vi "configure.vi"(8 "error in (no error)":errorcluster, 9 "write enable":bool=TRUE, 11 "SMSD in":refnum<class "SMSD.lvclass">) -> (0 "error out":errorcluster, 3 "SMSD out":refnum<class "SMSD.lvclass">)   [LabVIEW 2021, in "SMSD.lvclass"]
uses:
  SMSD.lvclass
  D:/my_projects/projects/Algorithms/Labview/21/Modbus/MB_TCP2/MB_TCP.lvclass
  SMSD.lvclass/SMSD.ctl
  Ctl/ERROR_OR_COMMANT_Type.ctl
  MB_TCP.lvclass/MB_TCP.ctl
  NI_modbus_upd/TCP/TCP.lvclass/TCP.ctl
  SMSD_cmd_format.vi
  NI_modbus_upd/TCP/Protocol Read.vi
  NI_modbus_upd/TCP/Protocol Write.vi
  Data Access/Read TCP.vi
  SMSD_cmd_Data_format.vi
  SMSD_LAN_COMMAND.vi
  <vilib>/Utility/error.llb/Clear Errors.vi
  NI_modbus_upd/TCP/TCP.lvclass
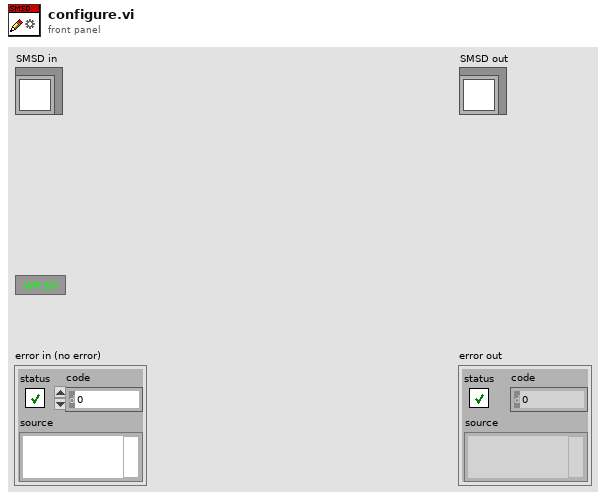
[diagram p1: front panel]
types:
  T1 = enum8{"CMD_PowerSTEP01_END", "CMD_PowerSTEP01_GET_SPEED", "CMD_PowerSTEP01_STATUS_IN_EVENT", "CMD_PowerSTEP01_SET_MODE", "CMD_PowerSTEP01_GET_MODE", "CMD_PowerSTEP01_SET_MIN_SPEED", "CMD_PowerSTEP01_SET_MAX_SPEED", "CMD_PowerSTEP01_SET_ACC", "CMD_PowerSTEP01_SET_DEC", "CMD_PowerSTEP01_SET_FS_SPEED", "CMD_PowerSTEP01_SET_MASK_EVENT", "CMD_PowerSTEP01_GET_ABS_POS", "CMD_PowerSTEP01_GET_EL_POS", "CMD_PowerSTEP01_GET_STATUS_AND_CLR", "CMD_PowerSTEP01_RUN_F", "CMD_PowerSTEP01_RUN_R", "CMD_PowerSTEP01_MOVE_F", "CMD_PowerSTEP01_MOVE_R", "CMD_PowerSTEP01_GO_TO_F", "CMD_PowerSTEP01_GO_TO_R", "CMD_PowerSTEP01_GO_UNTIL_F", "CMD_PowerSTEP01_GO_UNTIL_R", "CMD_PowerSTEP01_SCAN_ZERO_F", "CMD_PowerSTEP01_SCAN_ZERO_R", "CMD_PowerSTEP01_SCAN_LABEL_F", "CMD_PowerSTEP01_SCAN_LABEL_R", "CMD_PowerSTEP01_GO_ZERO", "CMD_PowerSTEP01_GO_LABEL", "CMD_PowerSTEP01_GO_TO", "CMD_PowerSTEP01_RESET_POS", "CMD_PowerSTEP01_RESET_POWERSTEP01", "CMD_PowerSTEP01_SOFT_STOP", "CMD_PowerSTEP01_HARD_STOP", "CMD_PowerSTEP01_SOFT_HI_Z", "CMD_PowerSTEP01_HARD_HI_Z", "CMD_PowerSTEP01_SET_WAIT", "CMD_PowerSTEP01_SET_RELE", "CMD_PowerSTEP01_CLR_RELE", "CMD_PowerSTEP01_GET_RELE", "CMD_PowerSTEP01_WAIT_IN0", "CMD_PowerSTEP01_WAIT_IN1", "CMD_PowerSTEP01_GOTO_PROGRAM", "CMD_PowerSTEP01_GOTO_PROGRAM_IF_IN0", "CMD_PowerSTEP01_GOTO_PROGRAM_IF_IN1", "CMD_PowerSTEP01_LOOP_PROGRAM", "CMD_PowerSTEP01_CALL_PROGRAM", "CMD_PowerSTEP01_RETURN_PROGRAM", "CMD_PowerSTEP01_START_PROGRAM_MEM0", "CMD_PowerSTEP01_START_PROGRAM_MEM1", "CMD_PowerSTEP01_START_PROGRAM_MEM2", "CMD_PowerSTEP01_START_PROGRAM_MEM3", "CMD_PowerSTEP01_STOP_PROGRAM_MEM", "CMD_PowerSTEP01_STEP_CLOCK", "CMD_PowerSTEP01_STOP_USB", "CMD_PowerSTEP01_GET_MIN_SPEED", "CMD_PowerSTEP01_GET_MAX_SPEED", "CMD_PowerSTEP01_GET_STACK", "CMD_PowerSTEP01_GOTO_PROGRAM_IF_ZERO", "CMD_PowerSTEP01_GOTO_PROGRAM_IF_IN_ZERO", "CMD_PowerSTEP01_WAIT_CONTINUE", "CMD_PowerSTEP01_SET_WAIT_2", "CMD_PowerSTEP01_SCAN_MARK2_F", "CMD_PowerSTEP01_SCAN_MARK2_R"}
  T2 = typedef "SMSD.lvclass/ERROR_OR_COMMANT_Type.ctl" = enum8{"OK", "OK_ACCESS", "ERROR_ACCESS", "ERROR_ACCESS_TIMEOUT", "ERROR_XOR", "ERROR_NO_COMMAND", "ERROR_LEN", "ERROR_RANGE", "ERROR_WRITE", "ERROR_READ", "ERROR_PROGRAMS", "ERROR_WRITE_SETUP", "NO_NEXT", "END_PROGRAMS", "COMMAND_GET_STATUS_IN_EVENT", "COMMAND_GET_MODE", "COMMAND_GET_ABS_POS", "COMMAND_GET_EL_POS", "COMMAND_GET_SPEED", "COMMAND_GET_MIN_SPEED", "COMMAND_GET_MAX_SPEED", "COMMAND_GET_STACK", "STATUS_RELE_SET", "STATUS_RELE_CLR"}
  T3 = cluster{"min_speed":u32, "max_speed":u32, "acc":u32, "dec":u32}
  T4 = typedef "SMSD.lvclass/MOTOR_PARAM.ctl" = cluster{"DRIVER_MODE":T5, "MOTOR_Type_42":T6, "MICROSTEPPING":T7, "WORK_CURRENT":T8, "STOP_CURRENT":T9}
  T5 = typedef "SMSD.lvclass/DRIVER_MODE.ctl" = enum16{"VOLTAGE", "CURRENT"}
  T6 = typedef "SMSD.lvclass/MOTOR_Type_42.ctl" = enum16{"Unknown", "FL42STH33-1334 1.8 deg", "FL42STH33-1334 0.9 deg", "FL42STH38-1206 0.9 deg", "FL42STH38-1684 1.8 deg", "FL42STH38-1684 0.9 deg", "FL42STH47-1206 1.8 deg", "FL42STH47-1684 1.8 deg", "FL42STH47-1684 0.9 deg", "FL42STH60-1206 1.8 deg", "FL42STH60-1206 0.9 deg", "FL57ST41-1564 1.8 deg", "FL57ST76-1006 1.8 deg", "FL57ST76-1506 1.8 deg", "FL57STH41-1006 1.8 deg", "FL57STH41-1006 0.9 deg", "FL57STH41-2804 1.8 deg", "FL57STH41-2804 0.9 deg", "FL57STH51-1006 1.8 deg", "FL57STH51-2804 1.8 deg", "FL57STH51-2804 0.9 deg", "FL57STH56-1006 1.8 deg", "FL57STH56-2006 1.8 deg", "FL57STH56-2804 1.8 deg", "FL57STH76-1006 1.8 deg", "FL57STH76-2804 1.8 deg", "FL57STH76-2804 0.9 deg", "FL60STH65-2008 1.8 deg parallel", "FL60STH65-2008 1.8 deg serial", "FL60STH86-2008 1.8 deg parallel", "FL60STH86-2008 1.8 deg serial", "FL86STH65-2808 1.8 deg parallel", "FL86STH65-2808 1.8 deg serial", "FL86STH80-4208 1.8 deg parallel", "FL86STH80-4208 1.8 deg serial", "FL86STH118-4208 1.8 deg parallel", "FL86STH118-4208 1.8 deg serial", "FL86STH156-4208 1.8 deg parallel", "FL86STH156-4208 1.8 deg serial", "ДШ3934-0,3А", "ДШ2851-0,7А", "ДШ4248-1,7A", "ДШ5776-3,0А", "ДШ57112-3,0А", "ДШ8665-3,0А", "ДШ8682-4,5А"}
  T7 = typedef "SMSD.lvclass/MICROSTEPPING.ctl" = enum16{"1", "1/2", "1/4", "1/8", "1/16", "1/32", "1/64", "1/128"}
  T8 = typedef "SMSD.lvclass/WORK_CURRENT.ctl" = enum16{"0.0A", "0.1A", "0.2A", "0.3A", "0.4A", "0.5A", "0.6A", "0.7A", "0.8A", "0.9A", "1.0A", "1.1A", "1.2A", "1.3A", "1.4A", "1.5A", "1.6A", "1.7A", "1.8A", "1.9A", "2.0A", "2.1A", "2.2A", "2.3A", "2.4A", "2.5A", "2.6A", "2.7A", "2.8A", "2.9A", "3.0A", "3.1A", "3.2A", "3.3A", "3.4A", "3.5A", "3.6A", "3.7A", "3.8A", "3.9A", "4.0A", "4.1A", "4.2A"}
  T9 = typedef "SMSD.lvclass/STOP_CURRENT.ctl" = enum16{"25%", "50%", "75%", "100%"}
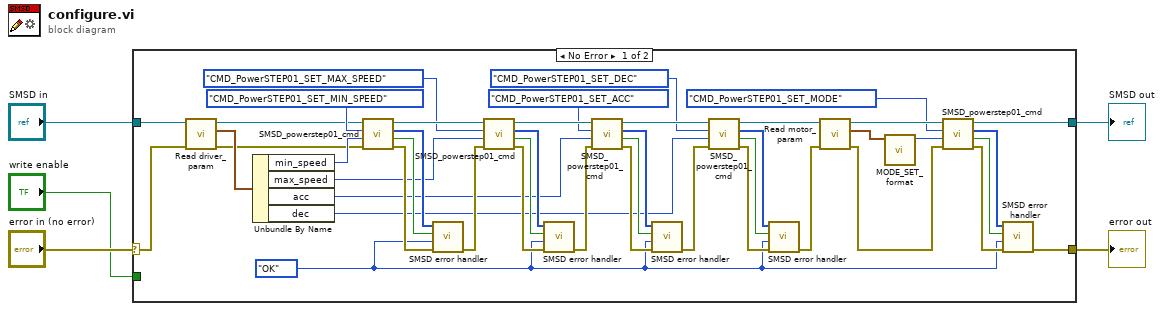
[diagram p0: block diagram]
diagram:
  n1 = case shown="No Error" "error in (no error)" {
    selector: "error in (no error)" -> [w6 w51]
    tunnel: [w12 w51] -> w3
    tunnel: [w10 w50] -> w4
    tunnel: "SMSD in" -> [w7 w50]
    tunnel: "write enable" -> [_ _]
    frame No Error {
      w11 = ERROR_OR_COMMANT_Type."OK" ("coerced x 2")
      n2 = call "Read driver_param.vi"("error in (no error)"=w6, "SMSD in"=w7) -> ("error out"=w45:errorcluster, "Driver_param"=w47:T3, "SMSD out"=w48:refnum<class "SMSD.lvclass">)  [unwired: 7 in]
      n3 = Unbundle By Name(w47) -> ("min_speed"=w46:u32, "max_speed"=w39:u32, "acc"=w29:u32, "dec"=w21:u32)
      n4 = call "SMSD_powerstep01_cmd.vi"("error in (no error)"=w45, "DATA (0)"=w46, "COMMAND (END)"=T1."CMD_PowerSTEP01_SET_MIN_SPEED", "SMSD in"=w48) -> ("error out"=w43:errorcluster, "timed out?"=w42:bool, "data"=w44:u8[], "SMSD out"=w41:refnum<class "SMSD.lvclass">)  [unwired: 4 in]
      n5 = call "SMSD error handler.vi"("error in (no error)"=w43, "correct answer (OK)"=w11, "timed out?"=w42, "data"=w44) -> ("error out"=w38:errorcluster)  [unwired: 7 in]
      n6 = call "SMSD_powerstep01_cmd.vi"("error in (no error)"=w38, "DATA (0)"=w39, "COMMAND (END)"=T1."CMD_PowerSTEP01_SET_MAX_SPEED", "SMSD in"=w41) -> ("error out"=w35:errorcluster, "timed out?"=w36:bool, "data"=w37:u8[], "SMSD out"=w30:refnum<class "SMSD.lvclass">)  [unwired: 4 in]
      n7 = call "SMSD error handler.vi"("error in (no error)"=w35, "correct answer (OK)"=w11, "timed out?"=w36, "data"=w37) -> ("error out"=w31:errorcluster)  [unwired: 7 in]
      n8 = call "SMSD_powerstep01_cmd.vi"("error in (no error)"=w31, "DATA (0)"=w29, "COMMAND (END)"=T1."CMD_PowerSTEP01_SET_ACC", "SMSD in"=w30) -> ("error out"=w34:errorcluster, "timed out?"=w33:bool, "data"=w32:u8[], "SMSD out"=w25:refnum<class "SMSD.lvclass">)  [unwired: 4 in]
      n9 = call "SMSD error handler.vi"("error in (no error)"=w34, "correct answer (OK)"=w11, "timed out?"=w33, "data"=w32) -> ("error out"=w24:errorcluster)  [unwired: 7 in]
      n10 = call "SMSD_powerstep01_cmd.vi"("error in (no error)"=w24, "DATA (0)"=w21, "COMMAND (END)"=T1."CMD_PowerSTEP01_SET_DEC", "SMSD in"=w25) -> ("error out"=w26:errorcluster, "timed out?"=w27:bool, "data"=w28:u8[], "SMSD out"=w20:refnum<class "SMSD.lvclass">)  [unwired: 4 in]
      n11 = call "SMSD error handler.vi"("error in (no error)"=w26, "correct answer (OK)"=w11, "timed out?"=w27, "data"=w28) -> ("error out"=w8:errorcluster)  [unwired: 7 in]
      n12 = call "Read motor_param.vi"("error in (no error)"=w8, "SMSD in"=w20) -> ("error out"=w9:errorcluster, "MOTOR_PARAM"=w19:T4, "SMSD out"=w15:refnum<class "SMSD.lvclass">)  [unwired: 7 in]
      n13 = call "MODE_SET_format.vi"("MOTOR_PARAM"=w19) -> ("Data"=w13:u32)  [unwired: 10 in]
      n14 = call "SMSD_powerstep01_cmd.vi"("error in (no error)"=w9, "DATA (0)"=w13, "COMMAND (END)"=T1."CMD_PowerSTEP01_SET_MODE", "SMSD in"=w15) -> ("error out"=w18:errorcluster, "timed out?"=w17:bool, "data"=w16:u8[], "SMSD out"=w10:refnum<class "SMSD.lvclass">)  [unwired: 4 in]
      n15 = call "SMSD error handler.vi"("error in (no error)"=w18, "correct answer (OK)"=w11, "timed out?"=w17, "data"=w16) -> ("error out"=w12:errorcluster)  [unwired: 7 in]
    }
    frame Error {
    }
  }
  "error out" <- w3
  "SMSD out" <- w4
